vi "CallExtract.vi"(6 "TracesRead error":errorcluster, 8 "VI folder":path, 10 "Pixmap.bin path":path, 11 "Traces.txt path":path) -> (2 "stderr":string, 3 "stdout":string, 4 "CallExtract error":errorcluster)   [LabVIEW 2023]
uses:
  <vilib>/Utility/error.llb/Trim Whitespace One-Sided.vi
panel:
  out "Input arguments":string
  out "Absolute paths":string
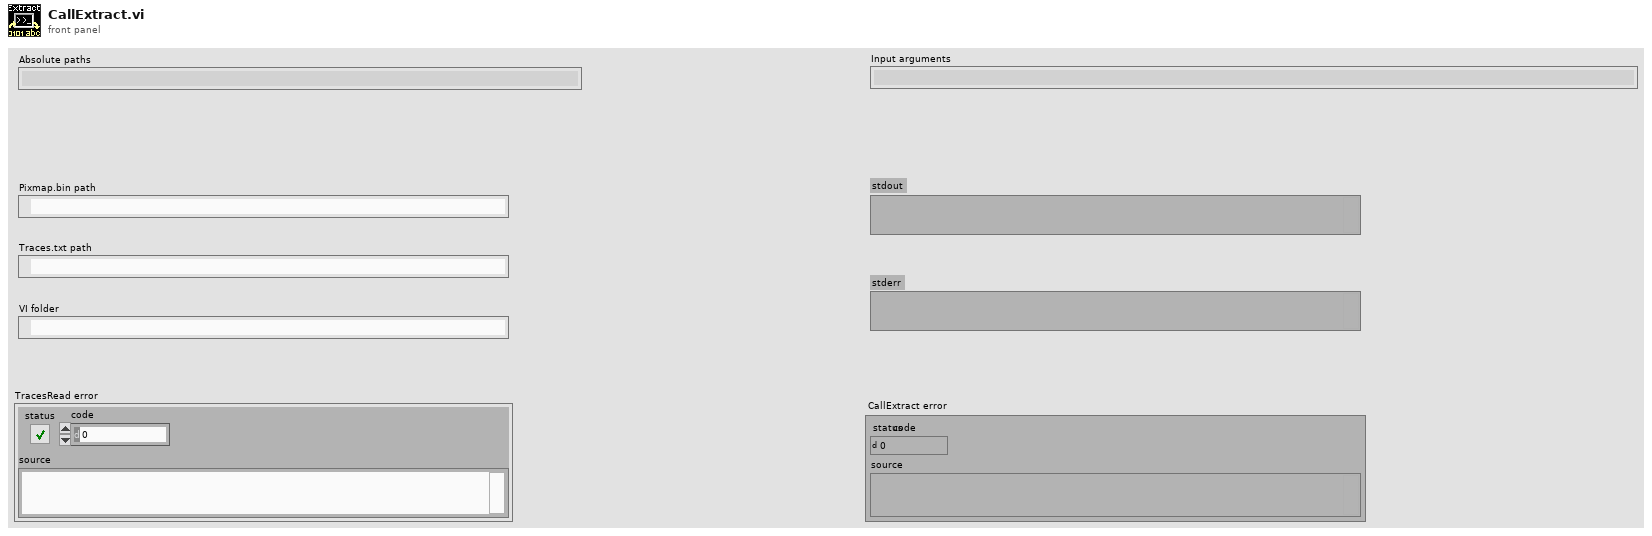
[diagram p1: front panel]
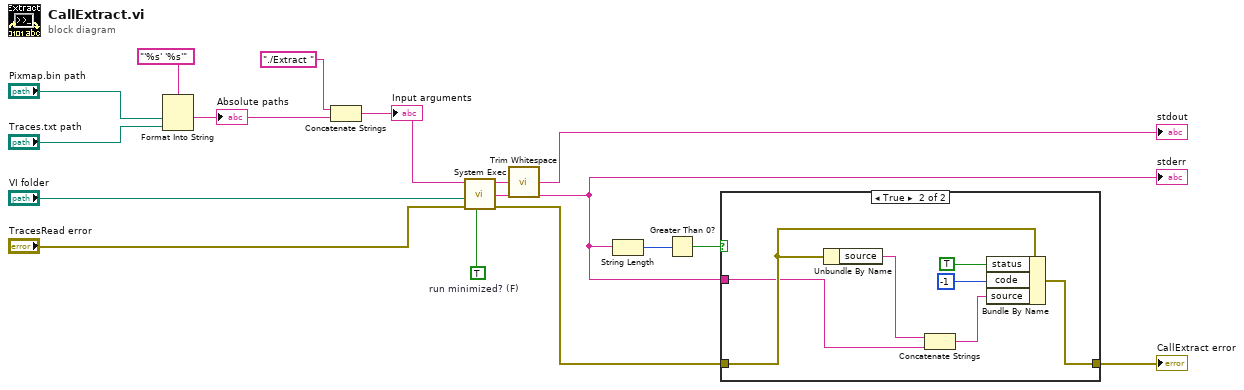
[diagram p0: block diagram]
diagram:
  w16 = TRUE  # run minimized? (F)
  n1 = Format Into String(format string="'%s' '%s'", "Pixmap.bin path", "Traces.txt path") -> (resulting string=w2:string)  [unwired: 2 in, 1 out]
  "Absolute paths" <- w2
  n2 = Concatenate Strings("./Extract " ("string"), w2) -> (w1:string)
  "Input arguments" <- w1
  n3 = call <vilib>:"System Exec.vi"("run minimized? (F)"=w16, "error in (no error)"="TracesRead error", "working directory"="VI folder", "command line"=w1) -> ("error out"=w7:errorcluster, "standard error"=w8:string, "standard output"=w12:string)  [unwired: 4 in, 1 out]
  "stderr" <- w8
  n4 = call <vilib>:"Trim Whitespace.vi"("string"=w12) -> ("trimmed string"=→"stdout":string)  [unwired: 1 in]
  n5 = String Length(string=w8) -> (length=w10:i32)
  n6 = Greater Than 0?(x=w10) -> (x > 0?=w9:bool)
  n7 = case shown="True" w9 {
    tunnel: w8 -> [_ w18]
    tunnel: w7 -> [w17 w23]
    tunnel: [w17 w24] -> w6
    frame False {
    }
    frame True {
      n8 = Unbundle By Name(w23) -> ("source"=w19:string)
      n9 = Concatenate Strings(w19, w18) -> (w20:string)
      n10 = Bundle By Name(cluster=w23, "status"=TRUE, "code"=-1, "source"=w20) -> (w24:errorcluster)
    }
  }
  "CallExtract error" <- w6
